vi "Read Supported Functions.vi"(8 "error in (no error)":errorcluster, 11 "Meter in":refnum<class "Meter.lvclass">) -> (0 "error out":errorcluster, 2 "Supported Functions":T1[](array[typedef]), 3 "Meter out":refnum<class "Meter.lvclass">)   [LabVIEW 2015, in "Meter.lvclass"]
uses:
  Meter.lvclass
  Mag Lab Hardware Function.ctl
  Mag Lab Hardware.lvclass
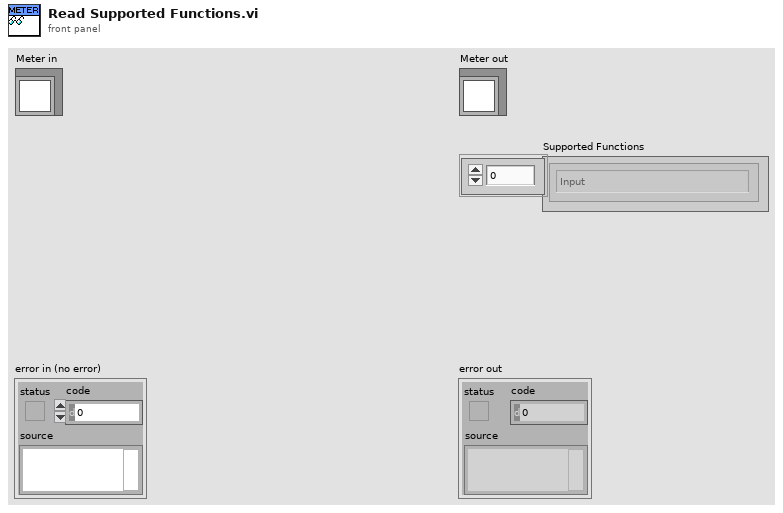
[diagram p1: front panel]
types:
  T1 = typedef "Mag Lab Hardware Function.ctl" = enum16{"Input", "Voltmeter", "Output", "Current source", "Digitizer", "Temperature controller"}
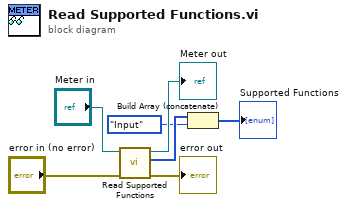
[diagram p0: block diagram]
diagram:
  n1 = call-parent "Read Supported Functions.vi"("error in (no error)"="error in (no error)", "Mag Lab Hardware in"="Meter in") -> ("error out"=→"error out":errorcluster, "Supported Functions"=w6:T1[], "Mag Lab Hardware out"=→"Meter out":refnum<class "Meter.lvclass">)  [unwired: 7 in]
  n2 = Build Array (concatenate)(w6, Mag_Lab_Hardware_Function."Input" ("Enum")) -> (→"Supported Functions":T1[])
